vi "Calculate Sweep ETA.vi"(9 "Target Field Rate (T/min)":dbl, 10 "Magnet Field (T)":dbl, 11 "Target Field (T)":dbl) -> (1 "Remaining Time (sec)":dbl, 2 "ETA string":string, 3 "ETA timestamp":timestamp)   [LabVIEW 2019, in "Instrument.OxfordVRM.lvclass"]
uses:
  Instrument.OxfordVRM.lvclass
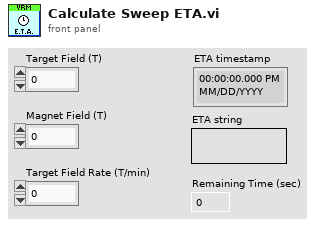
[diagram p1: front panel]
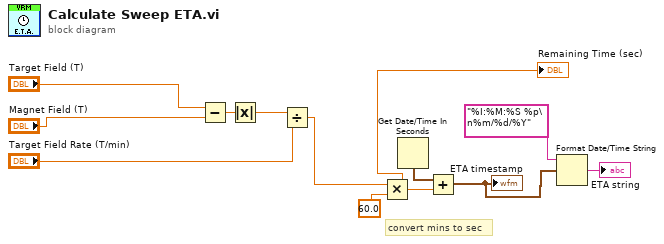
[diagram p0: block diagram]
diagram:
  # "convert mins to sec"
  n1 = Subtract(x="Target Field (T)", y="Magnet Field (T)") -> (x-y=w9:dbl)
  n2 = Absolute Value(x=w9) -> (abs(x)=w5:dbl)
  n3 = Divide(x=w5, y="Target Field Rate (T/min)") -> (x/y=w12:dbl)
  n4 = Multiply(x=w12, y=60.0 ("f")) -> (x*y=w4:dbl)
  "Remaining Time (sec)" <- w4
  n5 = Get Date/Time In Seconds() -> (seconds since 1Jan1904=w8:timestamp)
  n6 = Add(x=w8, y=w4) -> (x+y=w1:timestamp)
  "ETA timestamp" <- w1
  n7 = Format Date/Time String(time format string (%c)="%I:%M:%S %p\n%m/%d/%Y", seconds (now)=w1) -> (date/time string=→"ETA string":string)  [unwired: 1 in]
